vi "MB Ethernet Slave Ingen.vi"() -> ()   [LabVIEW 2017]
uses:
  NI Modbus.llb/MB Slave Init (poly).vi
  NI Modbus.llb/MB Globals.vi
  NI Modbus.llb/MB Slave Read All Coils (poly).vi
  NI Modbus.llb/MB Slave Read Holding Registers (poly).vi
  NI Modbus.llb/MB Slave Write Holding Registers (poly).vi
  NI Modbus.llb/MB Slave Write Discrete Inputs (poly).vi
panel:
  out "Input Registers":u16[](array[numeric])
  in  "Discrete Inputs (Master can only read these)":bool[](array[boolean])=[FALSE, FALSE, FALSE, FALSE]
  out "Consumo eléctrico Isla Numblar":u16[](array[numeric])
  in  "Listening Port":u16=502
  in  "Stop":bool
  out "Holding Registers":u16[](array[numeric]) caption="Holding Registers (Master can write in these registers)"
  out "Coils":bool[](array[boolean]) caption="Coils (Master can write coils)"
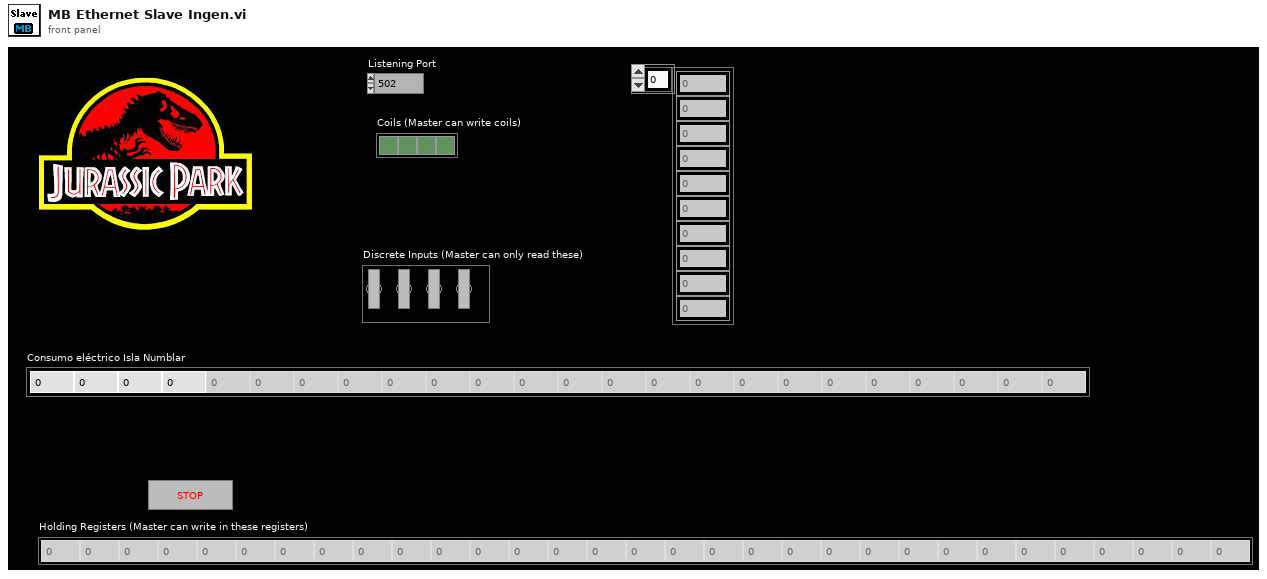
[diagram p1: front panel]
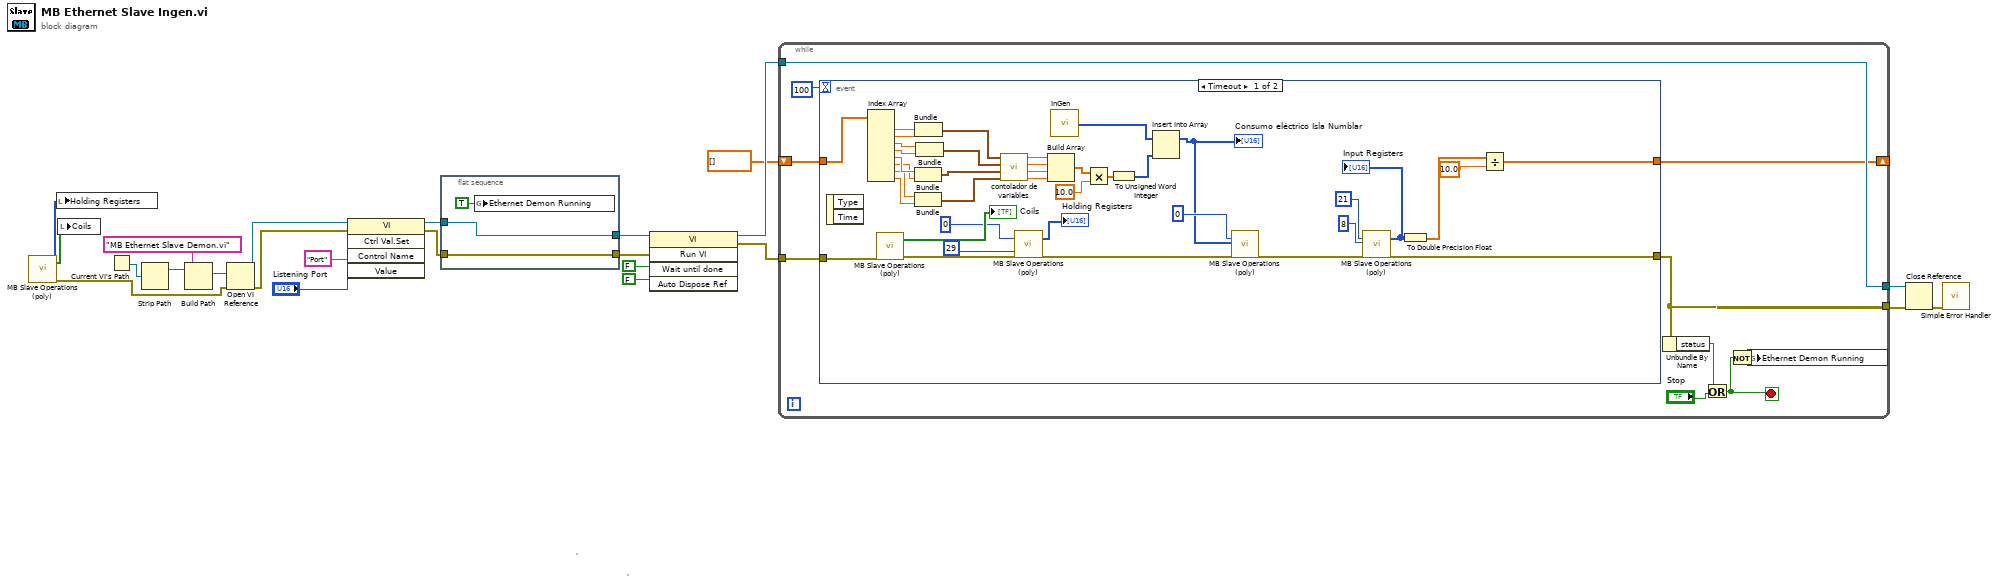
[diagram p0: block diagram]
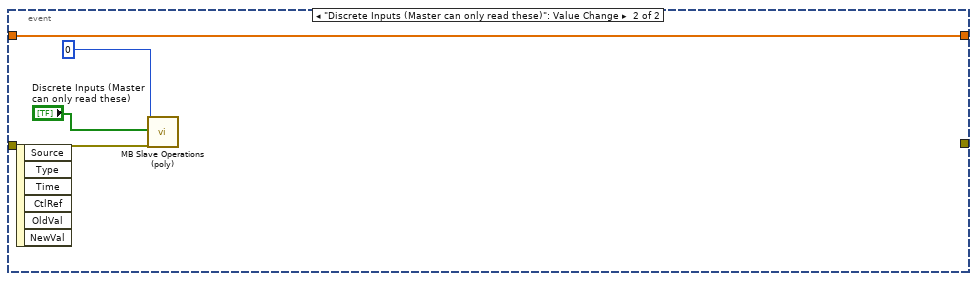
[diagram p2: hidden frame]
diagram:
  n1 = call-poly "MB Slave Operations (poly).vi"() -> ("Holding Registers"=w23:u16[], "Coils"=w6:bool[], "error out"=w9:errorcluster)  [unwired: 1 in, 16 out]
  n2 = local write "Holding Registers"(w23) -> ()
  n3 = local write "Coils"(w6) -> ()
  n4 = Current VI's Path() -> (path=w19:path)
  n5 = Strip Path(path=w19) -> (stripped path=w20:path)  [unwired: 1 out]
  n6 = Build Path(base path=w20, name or relative path="MB Ethernet Slave Demon.vi") -> (appended path=w22:path)
  n7 = Open VI Reference(vi path=w22, error in (no error)=w9) -> (vi reference=w16:refnum<vi>, error out=w15:errorcluster)  [unwired: 4 out]
  n8 = invoke class="VI" method="Ctrl Val.Set"(reference=w16, error in=w15, "Control Name"="Port", "Value"="Listening Port") -> (reference out=w2:refnum<vi>, error out=w3:errorcluster)  [unwired: 1 in, 3 out]
  n9 = flat-sequence {
    tunnel: [w26] -> w8
    tunnel: w3 -> [w26]
    tunnel: [w24] -> w5
    tunnel: w2 -> [w24]
    frame #0 {
      n10 = global write "MB Globals.vi" "Ethernet Demon Running"(TRUE ("Slave Demon Running")) -> ()
    }
  }
  n11 = invoke class="VI" method="Run VI"(reference=w5, error in=w8, "Wait until done"=FALSE, "Auto Dispose Ref"=FALSE) -> (reference out=w11:refnum<vi>, error out=w7:errorcluster)  [unwired: 1 in, 3 out]
  n12 = while {
    tunnel: [w31] -> w12
    tunnel: w11 -> [w31]
    tunnel: [w30] -> w10
    tunnel: w7 -> [w29]
    shift-right: [w28] -> _
    shift-left: dbl[] [] -> [w27]
    stop <- w32 stop-if-true
    n13 = event shown="[0] Timeout" {
      selector: _ -> [_ _]
      dyn-events: _ -> [_ _]
      timeout: 100 -> [_ _]
      tunnel: w29 -> [w75 w79]
      tunnel: [w40 _] -> w30
      tunnel: [w54 w76] -> w28
      tunnel: w27 -> [w53 w76]
      event Timeout {
        n14 = event-data() -> ()  [unwired: 3 out]
        n15 = Index Array "Index Array"(array=w53) -> (element #1=w52:dbl, element #2=w51:dbl, element #3=w50:dbl, element #4=w49:dbl, element #5=w48:dbl, element #6=w47:dbl, element #7=w46:dbl, element #8=w45:dbl)  [unwired: 8 in]
        n16 = call-poly "MB Slave Operations (poly).vi"("error in"=w75) -> ("Coils"=→"Coils":bool[], "error out"=w73:errorcluster)  [unwired: 17 out]
        n17 = Bundle(w48, w47) -> (w42:cluster{dbl, dbl})  [unwired: 1 in]
        n18 = Bundle(w46, w45) -> (w41:cluster{dbl, dbl})  [unwired: 1 in]
        n19 = Bundle(w52, w51) -> (w44:cluster{dbl, dbl})  [unwired: 1 in]
        n20 = Bundle(w50, w49) -> (w43:cluster{dbl, dbl})  [unwired: 1 in]
        n21 = call "contolador de variables.vi"("CONTROL DE LLENADO"=w41, "CONTROL DE HUMEDAD"=w42, "CONTROL DE PRESIÓN"=w43, "CONTROL TEMPERATURA"=w44) -> ("VOLUMEN ACTUAL"=w67:dbl, "HUMEDAD ACTUAL"=w68:dbl, "PRESIÓN ACTUAL"=w69:dbl, "TEMPERATURA ACTUAL"=w70:dbl)  [unwired: 4 in]
        n22 = call-poly "MB Slave Operations (poly).vi"("Starting Address"=u16 0, "Quantity"=u16 29, "error in"=w73) -> ("Holding Registers"=→"Holding Registers":u16[], "error out"=w71:errorcluster)  [unwired: 15 out]
        n23 = Build Array "Build Array"(w70, w69, w68, w67) -> (w66:dbl[])
        n24 = call "InGen.vi"() -> ("Variables de planta"=w63:u16[])
        n25 = Multiply(x=w66, y=10.0 ("VOLUMEN ACTUAL")) -> (x*y=w64:dbl[])
        n26 = To Unsigned Word Integer(number=w64) -> (unsigned 16bit integer=w62:u16[])
        n27 = Insert Into Array "Insert Into Array"(array=w63, new element=w62) -> (w61:u16[])  [unwired: 1 in]
        "Consumo eléctrico Isla Numblar" <- w61
        n28 = call-poly "MB Slave Operations (poly).vi"("Starting Address"=u16 0 ("Address"), "Holding Registers"=w61, "error in"=w71) -> ("error out"=w59:errorcluster)  [unwired: 1 in, 15 out]
        n29 = call-poly "MB Slave Operations (poly).vi"("Starting Address"=u16 21, "Quantity"=u16 8, "error in"=w59) -> ("Holding Registers"=w39:u16[], "error out"=w40:errorcluster)  [unwired: 1 in, 14 out]
        "Input Registers" <- w39
        n30 = To Double Precision Float(number=w39) -> (double precision float=w56:dbl[])
        n31 = Divide(x=w56, y=10.0) -> (x/y=w54:dbl[])
      }
      event "Discrete Inputs (Master can only read these)": Value Change {
        n32 = event-data() -> ()  [unwired: 7 out]
        n33 = call-poly "MB Slave Operations (poly).vi"("Starting Address"=u16 0, "Discrete Inputs"="Discrete Inputs (Master can only read these)", "error in"=w79) -> ()  [unwired: 1 in, 16 out]
      }
    }
    n34 = Unbundle By Name(w30) -> ("status"=w35:bool)
    n35 = Or(x=w35, y="Stop") -> (x .or. y?=w32:bool)
    n36 = Not(x=w32) -> (.not. x?=w33:bool)
    n37 = global write "MB Globals.vi" "Ethernet Demon Running"(w33) -> ()
  }
  n38 = Close Reference(reference=w12, error in (no error)=w10) -> (error out=w4:errorcluster)
  n39 = call <vilib>:"Simple Error Handler.vi"("error in (no error)"=w4) -> ()  [unwired: 1 in, 8 out]
